vi "save_infos_v4.vi"(0 "STAGE PORT":refnum<visa-resource-name>, 2 "info Directory":path, 3 "USED_FILTERS":u8[](array[numeric]), 5 "NB_CHANELS":u32, 6 "STAGE_SPEED":dbl, 7 "Noff_fluidix":u32, 8 "Camera infos":string, 9 "NUM_POS":u32, 10 "ROMODE":u32, 11 "Non_fluidix":u32, 12 "BIN":u16, 13 "NSCAN":u32, 14 "SOFT_VERSION":string, 15 "Nstart_fluidics":u32, 16 "EXPT":dbl, 17 "BETWEEN_SCAN":u32, 18 "USED_LEDS":bool[][](array[boolean]), 19 "useFLUIDCS":bool, 20 "Noff_laser":u32, 21 "Non_laser":u32, 22 "Nstart_laser":u32, 23 "BETWEEN_PATTERN":u32, 24 "NPATTERN":u32, 25 "is_singleshoot":bool, 26 "MIN SCAN DURATION":dbl, 27 "useLASER":bool) -> ()   [LabVIEW 2013]
panel:
  in  "SHOOT_AT_SCAN":u32
  in  "SHOOT_DUR":dbl
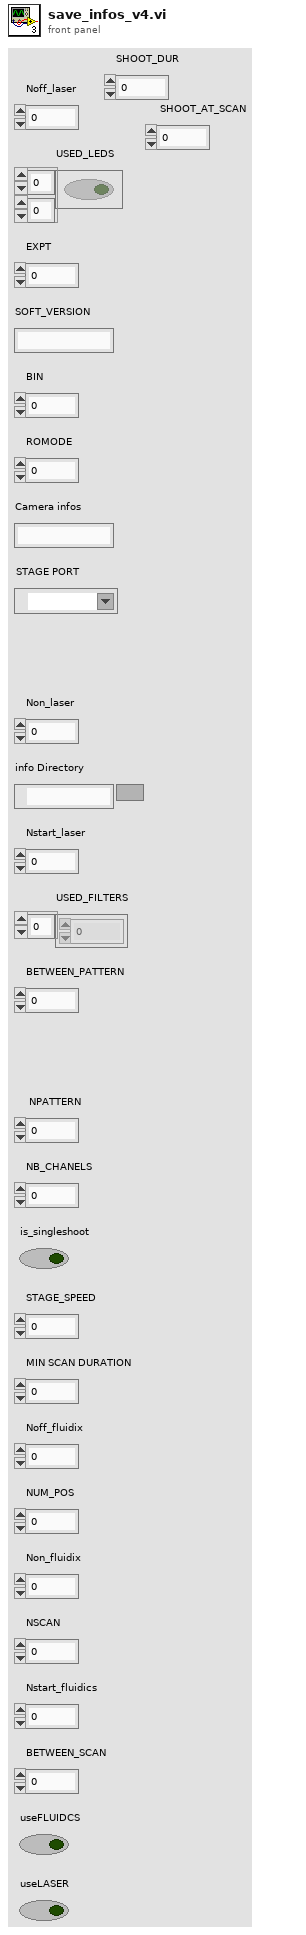
[diagram p1: front panel]
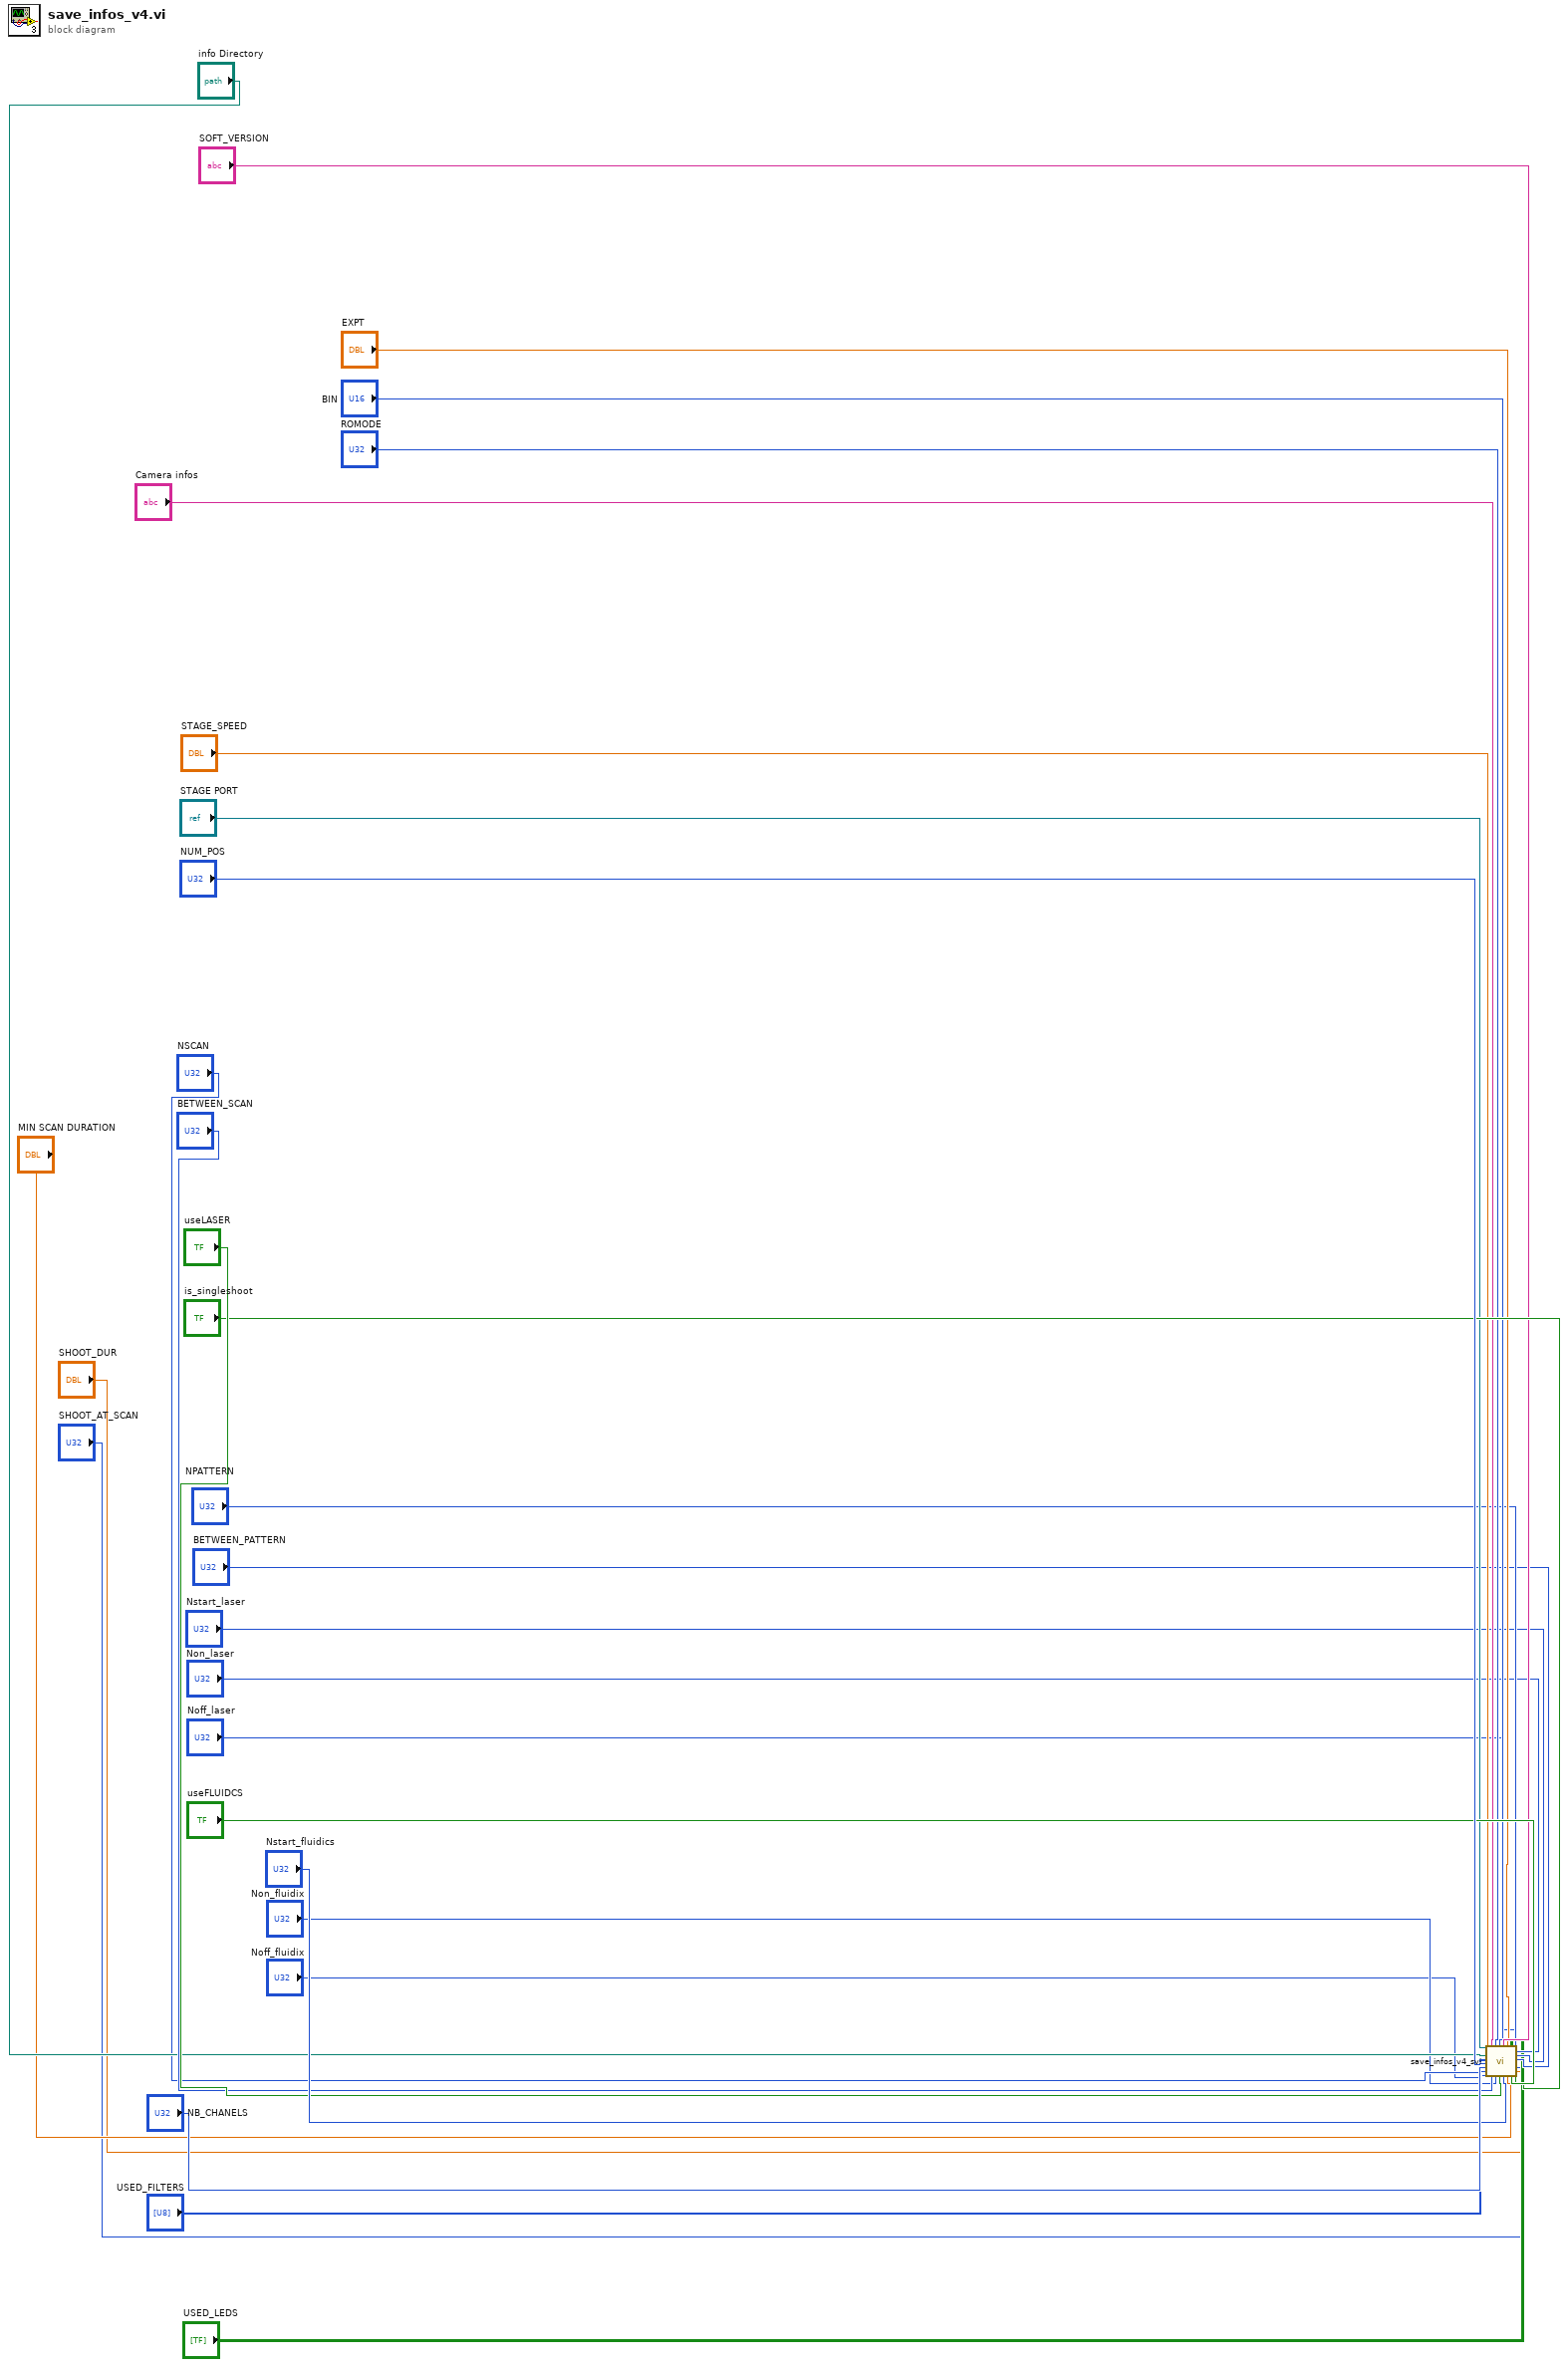
[diagram p0: block diagram]
diagram:
  n1 = call "save_infos_v4_svi.vi"("Refnum VISA en entrée"="STAGE PORT", "STAGE_SPEED"="STAGE_SPEED", "info Directory"="info Directory", "USED_FILTERS"="USED_FILTERS", "NUM_POS"="NUM_POS", "NB_CHANELS"="NB_CHANELS", "NSCAN"="NSCAN", "Noff_fluidix"="Noff_fluidix", "Camera infos"="Camera infos", "BETWEEN_SCAN"="BETWEEN_SCAN", "ROMODE"="ROMODE", "Non_fluidix"="Non_fluidix", "BIN"="BIN", "useLASER"="useLASER", "SOFT_VERSION"="SOFT_VERSION", "Nstart_fluidics"="Nstart_fluidics", "EXPT"="EXPT", "MIN SCAN DURATION"="MIN SCAN DURATION", "USED_LEDS"="USED_LEDS", "useFLUIDCS"="useFLUIDCS", "Noff_laser"="Noff_laser", "Non_laser"="Non_laser", "Nstart_laser"="Nstart_laser", "BETWEEN_PATTERN"="BETWEEN_PATTERN", "NPATTERN"="NPATTERN", "SHOOT_AT_SCAN"="SHOOT_AT_SCAN", "SHOOT_DUR"="SHOOT_DUR", "is_singleshoot"="is_singleshoot") -> ()
